vi "Help.vi"(5 "Point":T13, 6 "XRef":refnum<vi>, 7 "State In":T14) -> (0 "Subitem Help Info":T1, 1 "Detailed Help Info":T10, 2 "Standard Help Info":T8, 3 "Use Subitem Help?":bool, 4 "Use Detailed Help?":bool)   [LabVIEW 2012, in "OpenG FilterArray.xnode"]
doc: "This ability VI defines the XNode's context help (CH) and online help (OH) behavior.\n \n Standard Help Info: Consists of a Description (an explanation of the XNode to appear in CH window), and Path and Tag to the OH compiled html file.\n Use Detailed Help?: Set to false to allow the default context help and online help to be built using only those fields in Standard Help Info. Set to true to specify, in Detailed Help Info, the context help image and terminals to be drawn in context help.\n Detailed Help Info: Consists of an Image to display to the CH window, the Bounds of this image, and the Terms to draw in the CH window for this Image.\n Use Subitem Help? and Subitem Help Info: Reserved for future use.\n \n This ability VI is called whenever the CH system calls needs to update the CH window, and on a right click (to get the OH Path and Tag). The CH system is guaranteed to update the CH window whenever any of the following replies is sent: UpdateHelp, UpdateImage, UpdateImageAndBounds, UpdateLabel, UpdateTerms.\n\nDefault behavior: None.\n\nThis ability does not provide UI and OS messages are not handled."
uses:
  OpenG FilterArray.xnode
  <vilib>/XNodeSupport/XNodeImage.ctl
  <vilib>/XNodeSupport/NI_XNodeSupport.lvlib
  <vilib>/XNodeSupport/XNodeInt.ctl
  <vilib>/XNodeSupport/XNodeRect32.ctl
  <vilib>/XNodeSupport/XNodeString.ctl
  <vilib>/XNodeSupport/XNodeVariant.ctl
  <vilib>/XNodeSupport/XNodeBool.ctl
  <vilib>/XNodeSupport/XNodeTerm.ctl
  <vilib>/XNodeSupport/XNodeTerms.ctl
  <vilib>/XNodeSupport/XNodeDetailedHelpInfo.ctl
  <vilib>/XNodeSupport/XNodePath.ctl
  <vilib>/XNodeSupport/XNodeStandardHelpInfo.ctl
  State.ctl
  <vilib>/XNodeSupport/XNodePoint.ctl
  <vilib>/XNodeSupport/XNodeSubitemHelpInfo.ctl
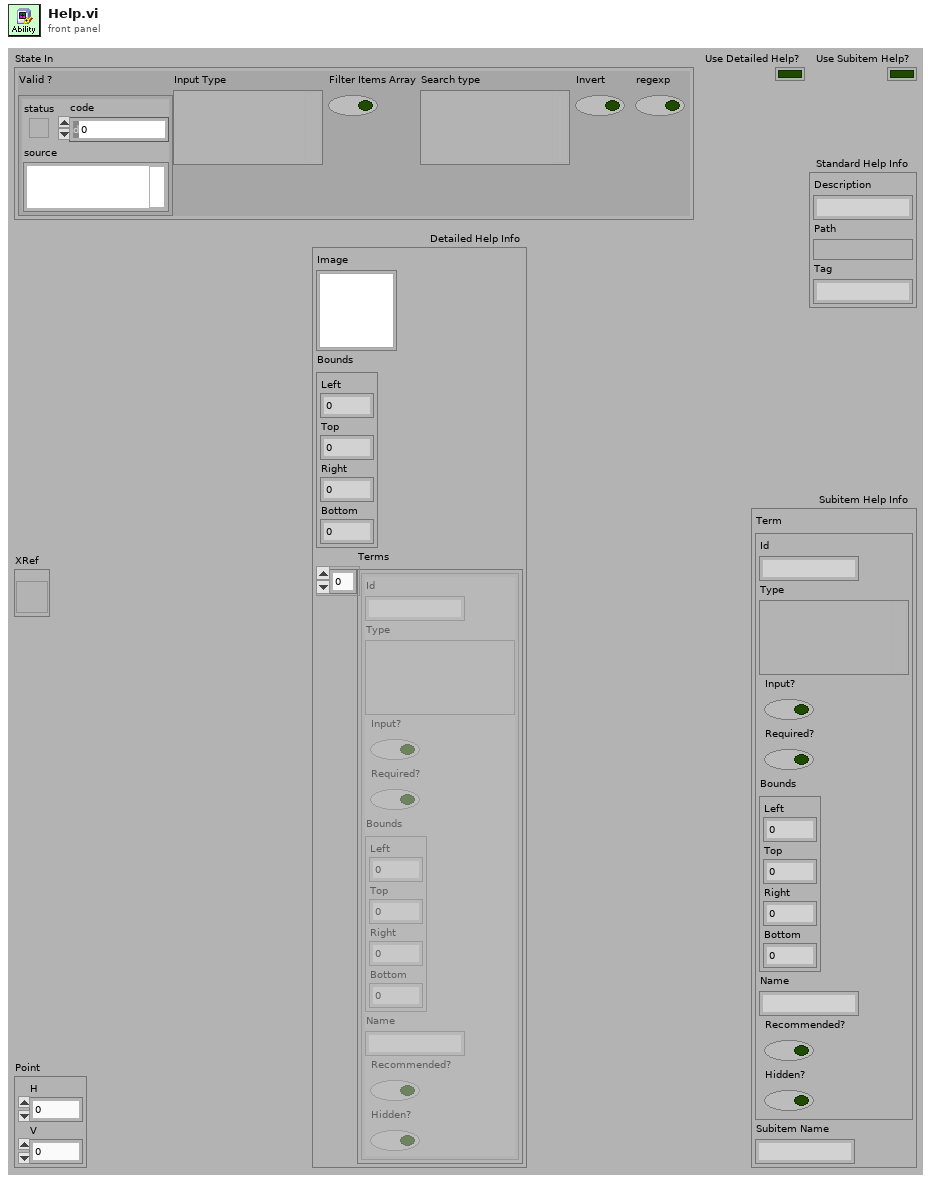
[diagram p1: front panel]
types:
  T1 = typedef "NI_XNodeSupport.lvlib/XNodeSubitemHelpInfo.ctl" = cluster{"Term":T2, "Subitem Name":T3}
  T2 = typedef "NI_XNodeSupport.lvlib/XNodeTerm.ctl" = cluster{"Id":T3, "Type":T4, "Input?":T5, "Required?":T5, "Bounds":T6, "Name":T3, "Recommended?":T5, "Hidden?":T5}
  T3 = typedef "NI_XNodeSupport.lvlib/XNodeString.ctl" = string
  T4 = typedef "NI_XNodeSupport.lvlib/XNodeVariant.ctl" = variant
  T5 = typedef "NI_XNodeSupport.lvlib/XNodeBool.ctl" = bool
  T6 = typedef "NI_XNodeSupport.lvlib/XNodeRect32.ctl" = cluster{"Left":T7, "Top":T7, "Right":T7, "Bottom":T7}
  T7 = typedef "NI_XNodeSupport.lvlib/XNodeInt.ctl" = i32
  T8 = typedef "NI_XNodeSupport.lvlib/XNodeStandardHelpInfo.ctl" = cluster{"Description":T3, "Path":T9, "Tag":T3}
  T9 = typedef "NI_XNodeSupport.lvlib/XNodePath.ctl" = path
  T10 = typedef "NI_XNodeSupport.lvlib/XNodeDetailedHelpInfo.ctl" = cluster{"Image":T11, "Bounds":T6, "Terms":T12}
  T11 = typedef "NI_XNodeSupport.lvlib/XNodeImage.ctl" = picture
  T12 = typedef "NI_XNodeSupport.lvlib/XNodeTerms.ctl" = T2[]
  T13 = typedef "NI_XNodeSupport.lvlib/XNodePoint.ctl" = cluster{"H":T7, "V":T7}
  T14 = typedef "OpenG FilterArray.xnode/State.ctl" = cluster{"Valid ?":errorcluster, "Input Type":variant, "Filter Items Array":bool, "Search type":variant, "Invert":bool, "regexp":bool}
  T15 = typedef "NI_XNodeSupport.lvlib/XNodeTerm3Array.ctl" = T16[]
  T16 = typedef "NI_XNodeSupport.lvlib/XNodeTerm3.ctl" = cluster{"Name":T3, "Id":T3, "Type":T4, "Bounds":T6, "Input?":T5, "Required?":T5, "Recommended?":T5, "Adaptive?":T5, "Hidden?":T5, "Direction":T17, "Break Wire?":T5}
  T17 = typedef "NI_XNodeSupport.lvlib/XNodeTermDirection.ctl" = enum32{"Auto", "Up", "Down", "Left", "Right", "Center"}
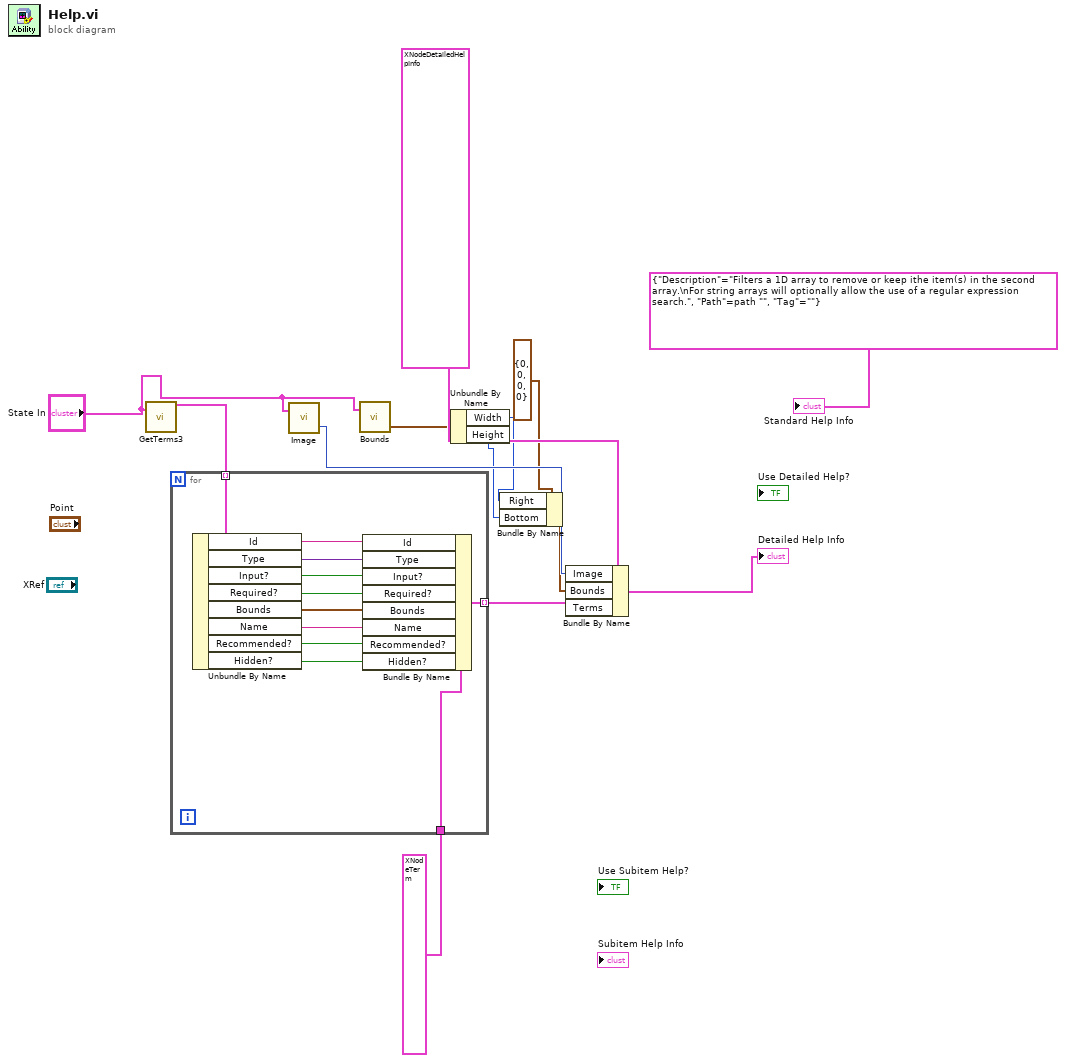
[diagram p0: block diagram]
diagram:
  n1 = call "GetTerms3.vi"("State In"="State In") -> ("Terms"=w12:T15)  [unwired: 1 in, 17 out]
  n2 = for {
    tunnel: T2 {"Id"="", "Type"=variant, "Input?"=FALSE, "Required?"=FALSE, "Bounds"={"Left"=0, "Top"=0, "Right"=0, "Bottom"=0}, "Name"="", "Recommended?"=FALSE, "Hidden?"=FALSE} ("Term") -> [w24]
    tunnel: w12 -> [w23] mode=indexing
    tunnel: [w14] -> w10 mode=indexing
    n3 = Unbundle By Name(w23) -> ("Id"=w22:T3, "Type"=w21:T4, "Input?"=w20:T5, "Required?"=w19:T5, "Bounds"=w18:T6, "Name"=w17:T3, "Recommended?"=w16:T5, "Hidden?"=w15:T5)
    n4 = Bundle By Name(cluster=w24, "Id"=w22, "Type"=w21, "Input?"=w20, "Required?"=w19, "Bounds"=w18, "Name"=w17, "Recommended?"=w16, "Hidden?"=w15) -> (w14:T2)
  }
  n5 = call "Image.vi"("State In"="State In") -> ("Image"=w8:picture)  [unwired: 1 in, 1 out]
  n6 = call "Bounds.vi"("State In"="State In") -> ("Bounds"=w5:cluster{"Width":T7, "Height":T7})  [unwired: 1 in]
  n7 = Unbundle By Name(w5) -> ("Width"=w4:T7, "Height"=w3:T7)
  n8 = Bundle By Name(cluster=T6 {"Left"=0, "Top"=0, "Right"=0, "Bottom"=0} ("Bounds"), "Right"=w4, "Bottom"=w3) -> (w2:T6)
  n9 = Bundle By Name(cluster=T10 {"Image"=bytes[0], "Bounds"={"Left"=0, "Top"=0, "Right"=0, "Bottom"=0}, "Terms"=[]} ("Detailed Help Info"), "Image"=w8, "Bounds"=w2, "Terms"=w10) -> (→"Detailed Help Info":T10)
  "Standard Help Info" <- T8 {"Description"="Filters a 1D array to remove or keep ithe item(s) in the second array.\nFor string arrays will optionally allow the use of a regular expression search.", "Path"=path "", "Tag"=""} ("Standard Help Info")
